vi "Telnet Close Connection.vi"(8 "error in (no error)":errorcluster, 11 "telnet connection":T1) -> (0 "error out":errorcluster, 3 "telnet connection out":T1)   [LabVIEW 2015, in "NI_InternetTK_Core_VIs.lvlib"]
doc: "Closes the connection associated with <B>telnet connection</B>."
uses:
  NI_InternetTK_Core_VIs.lvlib
  Telnet Session.ctl
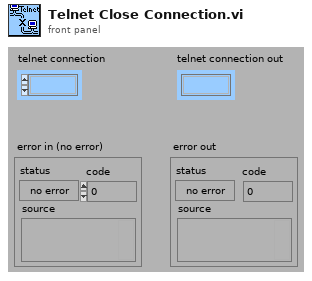
[diagram p1: front panel]
types:
  T1 = typedef "Telnet Session.ctl" = refnum<k1>
  T2 = enum16{"reset", "register", "get data", "set data", "unregister", "test", "get objects"}
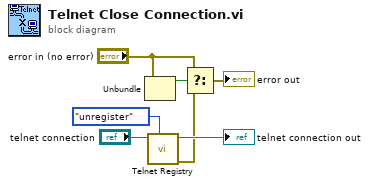
[diagram p0: block diagram]
diagram:
  n1 = Unbundle("error in (no error)") -> ("status"=w5:bool)  [unwired: 2 out]
  n2 = call "Telnet Registry.vi"("function (get data)"=T2."unregister", "object"="telnet connection") -> ("error out"=w3:errorcluster, "object out"=→"telnet connection out":T1)  [unwired: 2 in, 6 out]
  n3 = Select(t="error in (no error)", s=w5, f=w3) -> (s? t:f=→"error out":errorcluster)
